vi "Main.vi"(11 "Module Admin":refnum<class "Delacor_lib_QMH_Module Admin.lvclass">) -> ()   [LabVIEW 2024, in "UIs Handler.lvlib"]
doc: "This template is based off of the Queued Message Handler design pattern and the Queued Message Handler project template that ships with LabVIEW.\n\nThe main difference is that the queue is private to this module and communication between modules is performed via Broadcast and Request events.\n\nRequest events are wrapped in public API methods and are handled in the Event Handling Loop (EHL) of this VI. Any module can register for Broadcast events sent by this module. The EHL generates messages based on user interface actions.\n\nThe Message Handling Loop (MHL) processes messages generated by the EHL, or by other messages. The messages are string values, so new messages can be added easily to the Message Cases case structure in the MHL. Each message cluster can also provide an optional value for Message Data, which is a variant that can be converted to whatever message-specific data is required.\n_____\nBased on DQMH Dev Tools: Project Template 7.1.0.1490."
uses:
  UIs Handler.lvlib
  <vilib>/Delacor/Delacor QMH/Libraries/Module Admin_class/Delacor_lib_QMH_Module Admin.lvclass
  Module Data--cluster.ctl
  Stop Argument--cluster.ctl
  <vilib>/Delacor/Delacor QMH/Libraries/Message Queue_class/Delacor_lib_QMH_Message Queue.lvclass/Delacor_lib_QMH_Message Queue.ctl
  <vilib>/Delacor/Delacor QMH/Libraries/Module Admin_class/Delacor_lib_QMH_Module Admin.lvclass/Delacor_lib_QMH_Module Admin.ctl
  Insert UI into subpanel Argument--cluster.ctl
  UIs/Select UI.ctl
  Start Counter Argument--cluster.ctl
  Save Counter Argument--cluster.ctl
  <vilib>/Utility/miscctls.llb/LVPointTypeDef.ctl
  <vilib>/numeric/Random Number (Range) DBL.vi
  d7337ac3-38f4-4494-95c6-09e6596b0280.vi
  <vilib>/GPower/Timing/Library/Elapsed/Elapsed_ms.vi
  <vilib>/Delacor/Delacor QMH/Libraries/Message Queue_class/Delacor_lib_QMH_Enqueue Message (Single).vi
  <vilib>/Delacor/Delacor QMH/Libraries/Module Admin_class/Delacor_lib_QMH_Get External Launch.vi
  UIs/Dashboard.vi
  UIs/MetaTabs.vi
  <vilib>/GPower/VILauncher/Library/Open/OpenByRefnumAndRunFP.vi
  <vilib>/Utility/file.llb/Application Directory.vi
  <userlib>/_MGI/File/MGI Create Directory Chain.vi
  <vilib>/Utility/file.llb/Write Delimited Spreadsheet (DBL).vi
  <vilib>/Delacor/Delacor QMH/Libraries/Message Queue_class/Delacor_lib_QMH_Message Queue.lvclass
  <vilib>/GPower/Timing/GPTiming.lvlib
  <vilib>/GPower/VILauncher/VILauncher.lvlib
panel:
  out "file path":path
  out "Elapsed time":i32 caption="Elapsed time [ms]"
  out "output cluster":T1
  out "Waveform Chart":T2(graph)
  out "error out":errorcluster
  out "Status":string
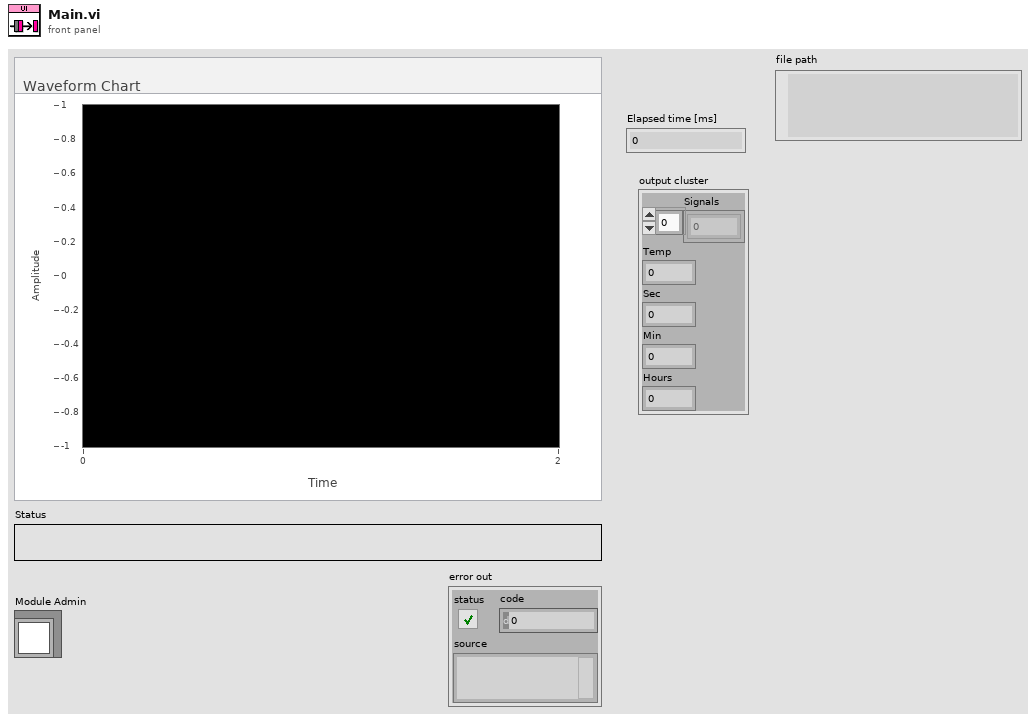
[diagram p1: front panel]
types:
  T1 = cluster{"Signals":dbl[], "Temp":dbl, "Sec":i32, "Min":i32, "Hours":i32}
  T2 = cluster{"shuffled array[0]":dbl, "shuffled array[1]":dbl, "shuffled array[2]":dbl, "shuffled array[3]":dbl, "shuffled array[4]":dbl, "shuffled array[5]":dbl, "shuffled array[6]":dbl, "shuffled array[7]":dbl, "shuffled array[8]":dbl, "shuffled array[9]":dbl, "shuffled array[10]":dbl, "shuffled array[11]":dbl, "shuffled array[12]":dbl, "shuffled array[13]":dbl, "shuffled array[14]":dbl, "shuffled array[15]":dbl, "shuffled array[16]":dbl, "shuffled array[17]":dbl, "shuffled array[18]":dbl, "shuffled array[19]":dbl}
  T3 = typedef "UIs Handler.lvlib/Request Events--cluster.ctl" = cluster{"Stop Module":refnum<user-event>, "Show Panel":refnum<user-event>, "Hide Panel":refnum<user-event>, "Get Module Execution Status":refnum<user-event>, "Show Diagram":refnum<user-event>, "Insert UI into subpanel":refnum<user-event>, "Start Counter":refnum<user-event>, "Reset Counter":refnum<user-event>, "Save Counter":refnum<user-event>, "Dashboard HLwakeup":refnum<user-event>, "Start Dashboard Monitoring":refnum<user-event>}
  T4 = typedef "UIs Handler.lvlib/Module Data--cluster.ctl" = cluster{"Status":string}
  T5 = cluster{"shuffled array[0]":dbl, "shuffled array[1]":dbl, "shuffled array[2]":dbl, "shuffled array[3]":dbl, "shuffled array[4]":dbl, "shuffled array[5]":dbl, "shuffled array[6]":dbl, "shuffled array[7]":dbl, "shuffled array[8]":dbl, "shuffled array[9]":dbl, "shuffled array[10]":dbl, "shuffled array[11]":dbl, "shuffled array[12]":dbl, "shuffled array[13]":dbl, "shuffled array[14]":dbl, "shuffled array[15]":dbl, "shuffled array[16]":dbl, "shuffled array[17]":dbl, "shuffled array[18]":dbl, "shuffled array[19]":dbl}[]
  T6 = enum32{"invalid lock state", "Not Locked", "Locked (No Password)", "Password-protected"}
  T7 = typedef "UIs Handler.lvlib/Stop Argument--cluster.ctl" = cluster{"Origin":string, "Exit via Stop Module Req?":bool, "Wait for Module to stop?":bool}
  T8 = typedef "UIs Handler.lvlib/Insert UI into subpanel Argument--cluster.ctl" = cluster{"Subpanel":refnum<vi>, "Select UI":T9}
  T9 = typedef "UIs Handler.lvlib/Select UI.ctl" = enum16{"Dashboard", "Meta Tabs"}
  T10 = typedef "UIs Handler.lvlib/Start Counter Argument--cluster.ctl" = cluster{"Boolean":bool}
  T11 = typedef "UIs Handler.lvlib/Save Counter Argument--cluster.ctl" = cluster{"Boolean":bool}
  T12 = typedef "LVPointTypeDef.ctl" = cluster{"Horizontal":i16, "Vertical":i16}
  T13 = enum32{"Invalid", "Standard", "Closed", "Hidden", "Minimized", "Maximized"}
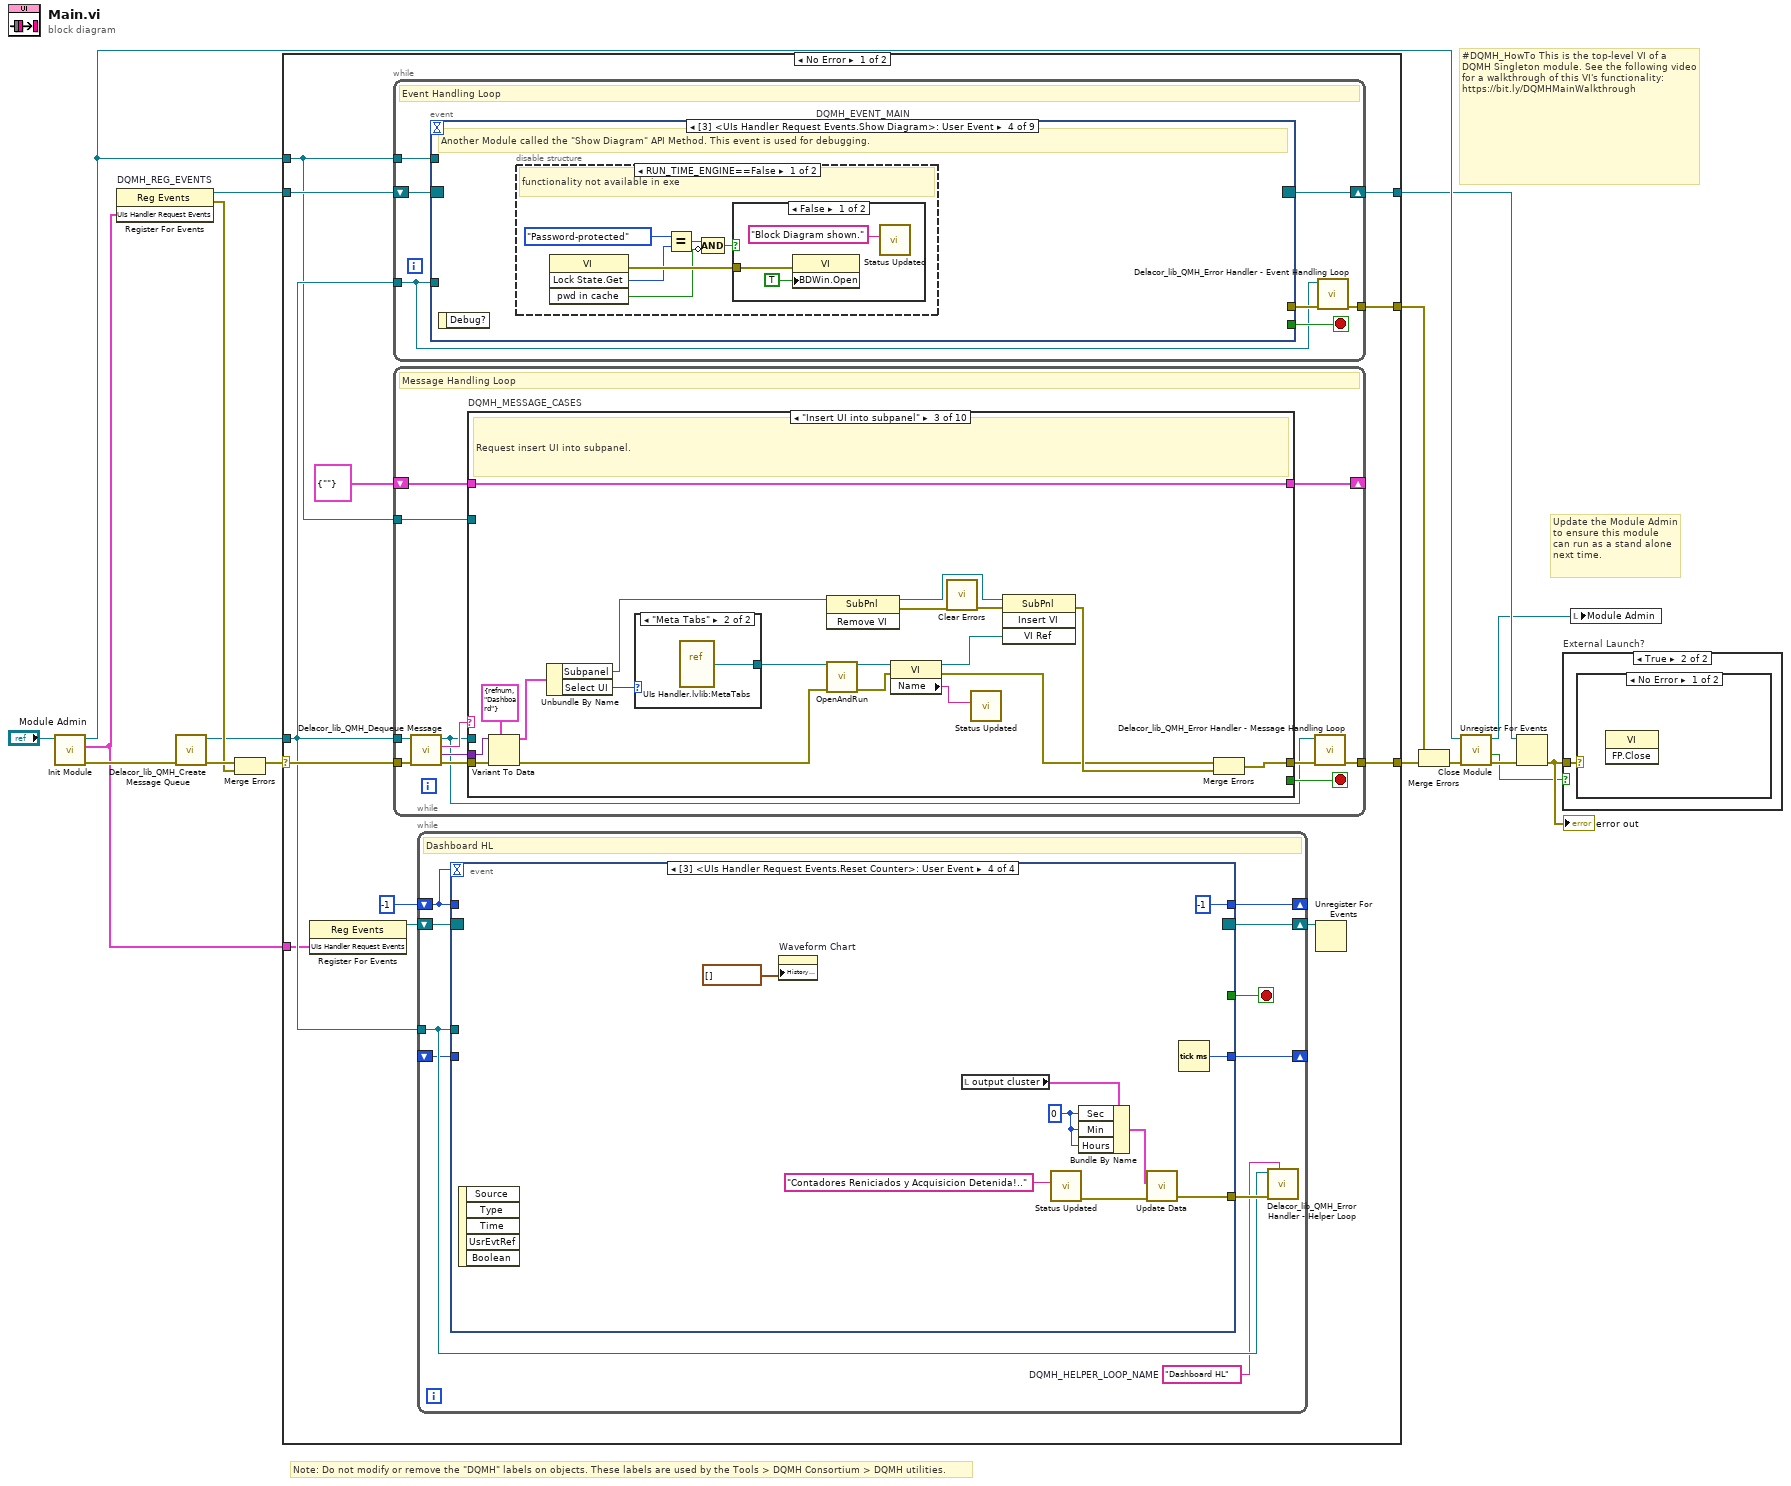
[diagram p0: block diagram]
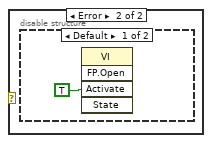
[diagram p3: hidden frame]
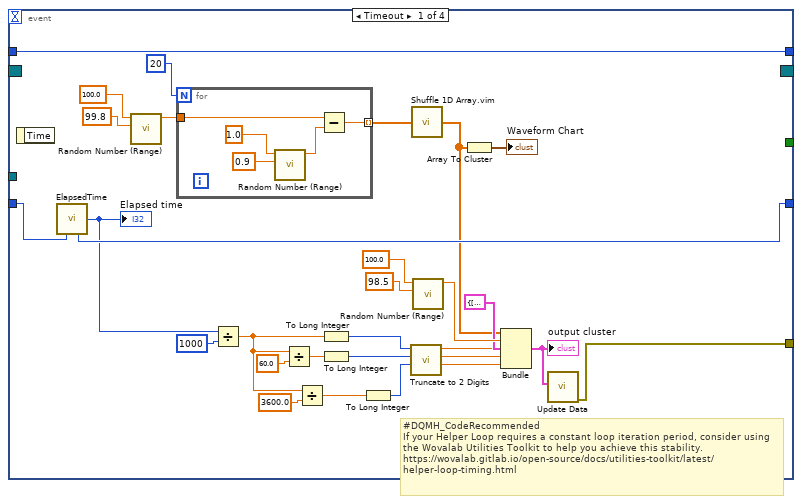
[diagram p5: hidden frame]
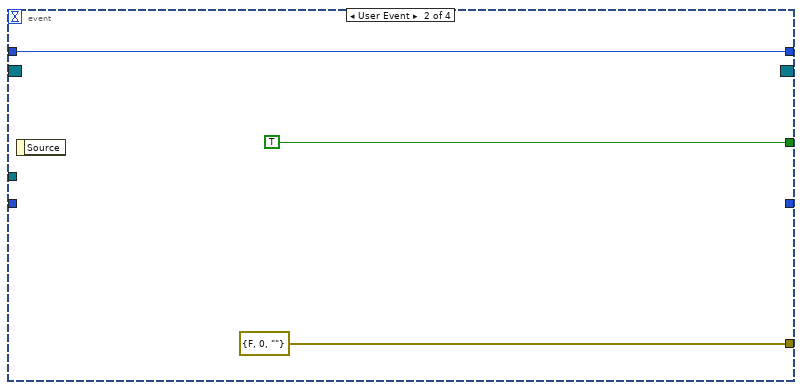
[diagram p6: hidden frame]
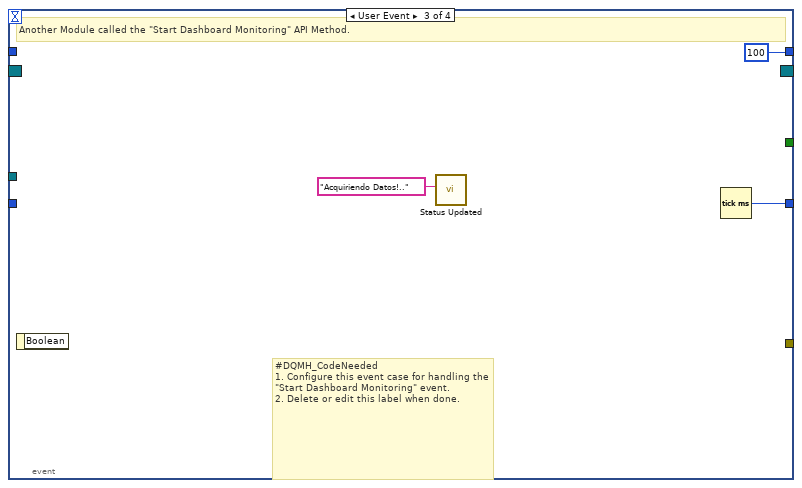
[diagram p7: hidden frame]
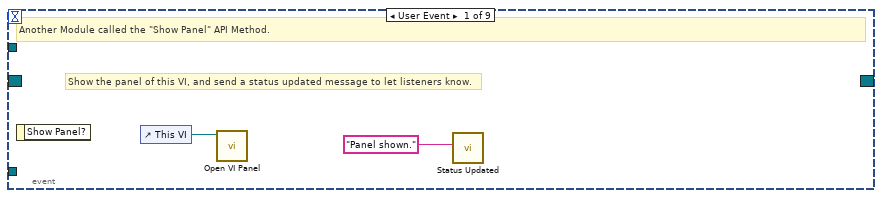
[diagram p8: hidden frame]
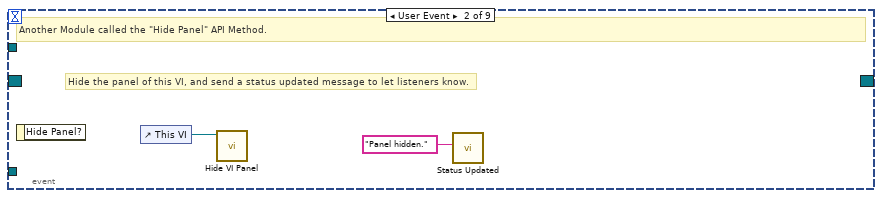
[diagram p9: hidden frame]
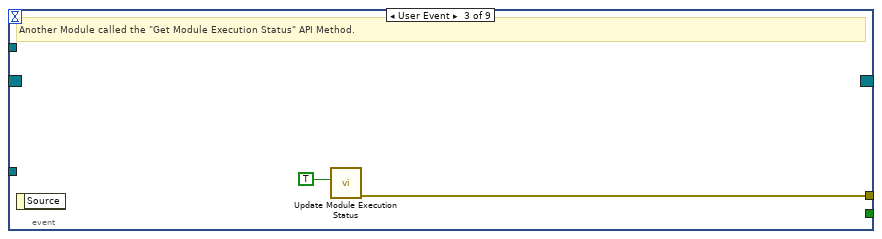
[diagram p10: hidden frame]
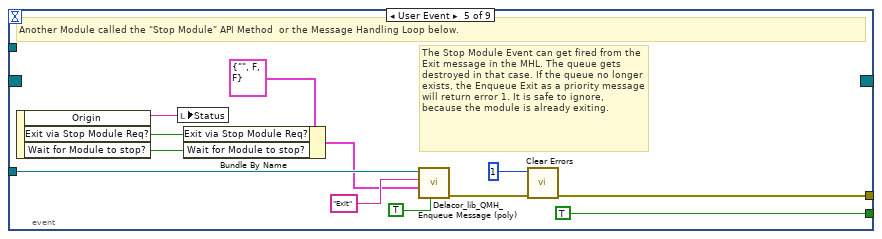
[diagram p13: hidden frame]
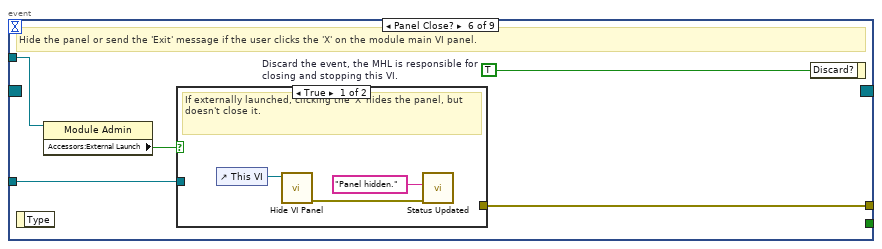
[diagram p14: hidden frame]
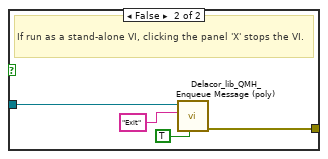
[diagram p15: hidden frame]
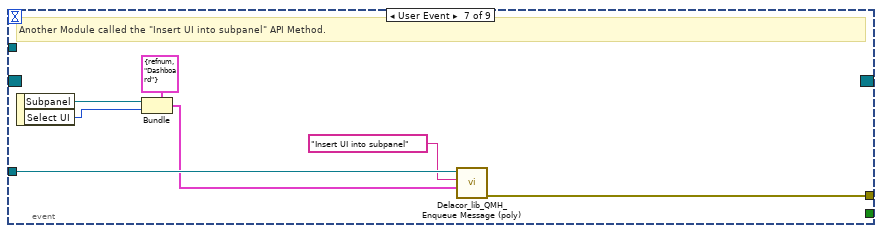
[diagram p16: hidden frame]
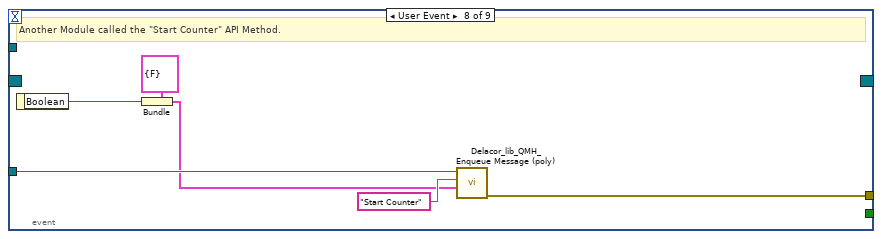
[diagram p17: hidden frame]
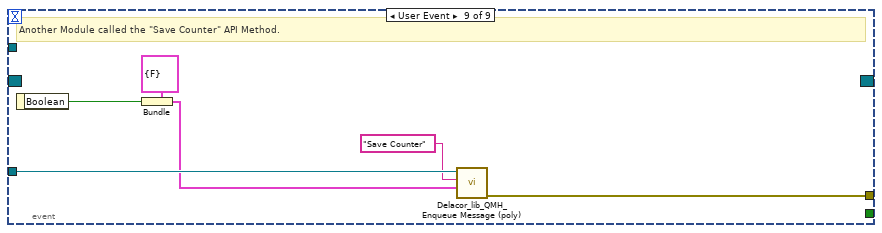
[diagram p18: hidden frame]
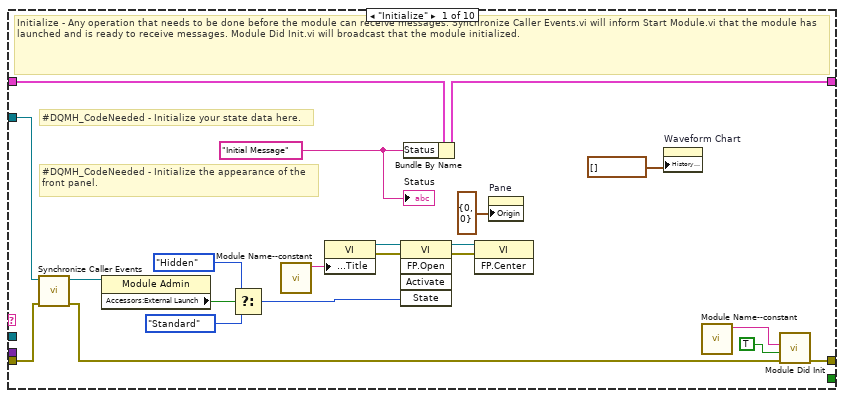
[diagram p19: hidden frame]
diagram:
  # "#DQMH_HowTo This is the top-level VI of a DQMH Singleton module. See the following video for a walkthrough of this VI's functionality: https://bit.ly/DQMHMainWalkthrough"
  # "Note: Do not modify or remove the \"DQMH\" labels on objects. These labels are used by the Tools > DQMH Consortium > DQMH utilities."
  # "Update the Module Admin to ensure this module can run as a stand alone next time."
  n1 = call "Init Module.vi"("Singleton Module Admin in"="Module Admin") -> ("error out"=w16:errorcluster, "UIs Handler Request Events"=w1:T3, "Singleton Module Admin out"=w8:refnum<class "Delacor_lib_QMH_Module Admin.lvclass">)  [unwired: 8 in]
  n2 = register-events "DQMH_REG_EVENTS"(w1) -> (reference out=w6:refnum<event-registration>, error out=w9:errorcluster)  [unwired: 2 in]
  n3 = call <vilib>:"Delacor_lib_QMH_Create Message Queue.vi"("error in"=w16) -> ("error out"=w11:errorcluster, "Message Queue"=w5:refnum<class "Delacor_lib_QMH_Message Queue.lvclass">)  [unwired: 9 in]
  n4 = Merge Errors(w11, w9) -> (w10:errorcluster)
  n5 = case shown="No Error" w10 {
    selector: w10 -> [w27 w288]
    tunnel: [w29 w287] -> w17
    tunnel: [w26 w286] -> w7
    tunnel: w6 -> [w24 w286]
    tunnel: w5 -> [w23 w281]
    tunnel: [w28 _] -> w14
    tunnel: w8 -> [w22 w282]
    tunnel: w1 -> [w21 _]
    frame No Error {
      n6 = register-events ("DQMH_HELPER_REGFOREVENTS")(w21) -> (reference out=w19:refnum<event-registration>)  [unwired: 2 in, 1 out]
      n7 = while {
        tunnel: w23 -> [w89]
        shift-right: [w92] -> w26
        shift-left: w24 -> [w93]
        tunnel: [w94] -> w28
        tunnel: w22 -> [w90]
        stop <- w91 stop-if-true
        # "Event Handling Loop"
        n8 = event "DQMH_EVENT_MAIN" shown="[3] <UIs Handler Request Events.Show Diagram>: User Event" {
          selector: w93 -> [_ _ _ _ _ _ _ _ _]
          dyn-events: [_ _ _ _ _ _ _ _ _] -> w92
          timeout: _ -> [_ _ _ _ _ _ _ _ _]
          tunnel: [_ _ _ _ TRUE ("Discard?") _ _ _ _] -> w91
          tunnel: w89 -> [_ _ _ _ w118 w125 w141 w147 w153]
          tunnel: [_ _ w101 _ w121 w127 w135 w142 w148] -> w95
          tunnel: w90 -> [_ _ _ _ _ w124 _ _ _]
          event User Event {
            # "Show the panel of this VI, and send a status updated message to let listeners know."
            # "Another Module called the \"Show Panel\" API Method."
            n9 = event-data() -> ()  [unwired: 1 in, 1 out]
            n10 = control-ref of="This VI"() -> (w97:refnum<vi>)
            n11 = call "Open VI Panel.vi"("VI"=w97) -> ()  [unwired: 10 in, 1 out]
            n12 = call "Status Updated.vi"("Status"="Panel shown." ("format string")) -> ()  [unwired: 10 in, 1 out]
          }
          event User Event {
            # "Hide the panel of this VI, and send a status updated message to let listeners know."
            # "Another Module called the \"Hide Panel\" API Method."
            n13 = event-data() -> ()  [unwired: 1 in, 1 out]
            n14 = control-ref of="This VI"() -> (w99:refnum<vi>)
            n15 = call "Hide VI Panel.vi"("VI"=w99) -> ()  [unwired: 10 in, 1 out]
            n16 = call "Status Updated.vi"("Status"="Panel hidden." ("format string")) -> ()  [unwired: 10 in, 1 out]
          }
          event User Event {
            # "Another Module called the \"Get Module Execution Status\" API Method."
            n17 = event-data() -> ()  [unwired: 1 in, 1 out]
            n18 = call "Update Module Execution Status.vi"("Running?"=TRUE) -> ("error out"=w101:errorcluster)  [unwired: 10 in]
          }
          event User Event {
            # "Another Module called the \"Show Diagram\" API Method. This event is used for debugging."
            n19 = event-data() -> ()  [unwired: 1 in, 1 out]
            n20 = disable-structure shown="RUN_TIME_ENGINE==False" {
              frame condition #0 (active) {
                # "functionality not available in exe"
                n21 = invoke on="Invoke Node" class="VI" method="Lock State.Get"() -> (error out=w107:errorcluster, "Get Lock State"=w106:T6, "pwd in cache"=w103:bool)  [unwired: 4 in, 1 out]
                n22 = Equal?(x=T6."Password-protected", y=w106) -> (x = y?=w104:bool)
                n23 = Compound Arithmetic op=AND(w104, invert w103) -> (w102:bool)
                n24 = case shown="False" w102 {
                  tunnel: w107 -> [w110 _]
                  frame False {
                    n25 = property on="Property Node" class="VI"(error in=w110, "BDWin.Open"=TRUE ("Block Diagram Window:Open")) -> ()  [unwired: 1 in, 2 out]
                    n26 = call "Status Updated.vi"("Status"="Block Diagram shown." ("format string")) -> ()  [unwired: 10 in, 1 out]
                  }
                  frame True {
                    # "Password-protected VI, and the password is not in the cache. Do not show the diagram."
                  }
                }
              }
              frame condition #1 {
              }
            }
          }
          event User Event {
            # "The Stop Module Event can get fired from the Exit message in the MHL. The queue gets destroyed in that case. If the queue no longer exists, the Enqueue Exit as a priority message will return error 1. It is safe to ignore, because the module is already exiting."
            # "Another Module called the \"Stop Module\" API Method  or the Message Handling Loop below."
            n27 = event-data() -> ("Origin"=w117:string, "Exit via Stop Module Req?"=w113:bool, "Wait for Module to stop?"=w112:bool)  [unwired: 1 in]
            n28 = local write "Status"(w117) -> ()
            n29 = Bundle By Name(cluster=T7 {"Origin"="", "Exit via Stop Module Req?"=FALSE, "Wait for Module to stop?"=FALSE} ("Stop Argument"), "Exit via Stop Module Req?"=w113, "Wait for Module to stop?"=w112) -> (w111:T7)
            n30 = call-poly <vilib>:"Delacor_lib_QMH_Enqueue Message (poly).vi"("Priority Message? (F)"=TRUE, "Message Data"=w111, "Message"="Exit", "Message Queue in"=w118) -> ("error out"=w122:errorcluster)  [unwired: 6 in, 1 out]
            n31 = call <vilib>:"Clear Errors.vi"("error in (no error)"=w122, "specific error code to clear (0: all)"=1) -> ("error out"=w121:errorcluster)  [unwired: 4 in, 1 out]
          }
          event Panel Close? {
            w126 = TRUE  # Discard the event, the MHL is responsible for closing and stopping this VI.
            # "Hide the panel or send the 'Exit' message if the user clicks the 'X' on the module main VI panel."
            n32 = event-data() -> ()  [unwired: 1 in, 1 out]
            n33 = property on="Property Node" class="Module Admin"(reference=w124) -> ("Accessors:External Launch"=w123:bool)  [unwired: 1 in, 2 out]
            n34 = case shown="True" w123 {
              tunnel: w125 -> [_ w133]
              tunnel: [_ w134] -> w127
              frame True {
                # "If externally launched, clicking the 'X' hides the panel, but doesn't close it."
                n35 = control-ref of="This VI"() -> (w130:refnum<vi>)
                n36 = call "Hide VI Panel.vi"("VI"=w130) -> ("error out"=w128:errorcluster)  [unwired: 10 in]
                n37 = call "Status Updated.vi"("error in"=w128, "Status"="Panel hidden." ("format string")) -> ()  [unwired: 9 in, 1 out]
              }
              frame False {
                # "If run as a stand-alone VI, clicking the panel 'X' stops the VI."
                n38 = call-poly <vilib>:"Delacor_lib_QMH_Enqueue Message (poly).vi"("Priority Message? (F)"=TRUE, "Message"="Exit", "Message Queue in"=w133) -> ("error out"=w134:errorcluster)  [unwired: 7 in, 1 out]
              }
            }
            n39 = event-data ("Event Filter Node")("Discard?"=w126) -> ()  [unwired: 1 in, 1 out]
          }
          event User Event {
            # "Another Module called the \"Insert UI into subpanel\" API Method."
            n40 = event-data() -> ("Subpanel"=w137:refnum<vi>, "Select UI"=w136:T9)  [unwired: 1 in]
            n41 = Bundle(cluster=T8 {"Subpanel"=refnum, "Select UI"=enum."Dashboard"} ("Insert UI into subpanel Argument"), "Subpanel"=w137, "Select UI"=w136) -> (w138:T8)
            n42 = call-poly <vilib>:"Delacor_lib_QMH_Enqueue Message (poly).vi"("Message Data"=w138, "Message"="Insert UI into subpanel", "Message Queue in"=w141) -> ("error out"=w135:errorcluster)  [unwired: 7 in, 1 out]
          }
          event User Event {
            # "Another Module called the \"Start Counter\" API Method."
            n43 = event-data() -> ("Boolean"=w143:bool)  [unwired: 1 in]
            n44 = Bundle(cluster=T10 {"Boolean"=FALSE} ("Start Counter Argument"), "Boolean"=w143) -> (w144:T10)
            n45 = call-poly <vilib>:"Delacor_lib_QMH_Enqueue Message (poly).vi"("Message Data"=w144, "Message"="Start Counter", "Message Queue in"=w147) -> ("error out"=w142:errorcluster)  [unwired: 7 in, 1 out]
          }
          event User Event {
            # "Another Module called the \"Save Counter\" API Method."
            n46 = event-data() -> ("Boolean"=w149:bool)  [unwired: 1 in]
            n47 = Bundle(cluster=T11 {"Boolean"=FALSE} ("Save Counter Argument"), "Boolean"=w149) -> (w150:T11)
            n48 = call-poly <vilib>:"Delacor_lib_QMH_Enqueue Message (poly).vi"("Message Data"=w150, "Message"="Save Counter", "Message Queue in"=w153) -> ("error out"=w148:errorcluster)  [unwired: 7 in, 1 out]
          }
        }
        n49 = call-dynamic "Delacor_lib_QMH_Error Handler - Event Handling Loop.vi"("error in"=w95, "Message Queue in"=w89) -> ("dup error in"=w94:errorcluster)  [unwired: 8 in, 1 out]
      }
      n50 = while {
        tunnel: w23 -> [w154]
        shift-right: [w162] -> _
        shift-left: T4 {"Status"=""} ("Data Cluster") -> [w163]
        tunnel: w27 -> [w165]
        tunnel: [w157] -> w29
        tunnel: w22 -> [w158]
        stop <- w161 stop-if-true
        # "Message Handling Loop"
        n51 = call-dynamic "Delacor_lib_QMH_Dequeue Message.vi"("error in"=w165, "Message Queue in"=w154) -> ("error out"=w164:errorcluster, "Message Data"=w159:variant, "Message"=w160:string, "Message Queue out"=w155:refnum<class "Delacor_lib_QMH_Message Queue.lvclass">)  [unwired: 6 in]
        n52 = case "DQMH_MESSAGE_CASES" shown="\"Insert UI into subpanel\"" w160 {
          selector: w160 -> [_ _ _ _ _ _ _ _ _ w276]
          tunnel: w155 -> [_ _ _ _ _ _ _ w242 w264 _]
          tunnel: w164 -> [w184 w188 w207 w217 w233 w236 w238 w249 w270 w279]
          tunnel: [w182 w188 w195 w210 w221 w235 w238 w245 w265 w280] -> w156
          tunnel: w163 -> [w173 w187 w206 w216 w232 w234 w237 w244 w263 w277]
          tunnel: [w172 w187 w206 w216 w232 w234 w237 w244 w263 w277] -> w162
          tunnel: [_ _ _ _ _ _ _ _ w262 _] -> w161
          tunnel: w159 -> [_ _ w205 w215 w231 _ _ w243 w261 _]
          tunnel: w158 -> [w174 _ _ _ _ _ _ w241 w256 _]
          frame "Initialize" {
            w168 = "Initial Message" ("Initial Message")
            # "#DQMH_CodeNeeded - Initialize the appearance of the front panel."
            # "#DQMH_CodeNeeded - Initialize your state data here."
            # "Initialize - Any operation that needs to be done before the module can receive messages. Synchronize Caller Events.vi will inform Start Module.vi that the module has launched and is ready to receive messages. Module Did Init.vi will broadcast that the module initialized."
            n53 = call "Synchronize Caller Events.vi"("error in"=w184, "Singleton Module Admin in"=w174) -> ("error out"=w183:errorcluster, "Singleton Module Admin out"=w169:refnum<class "Delacor_lib_QMH_Module Admin.lvclass">)  [unwired: 8 in]
            n54 = property on="Property Node" class="Module Admin"(reference=w169) -> ("Accessors:External Launch"=w178:bool)  [unwired: 1 in, 2 out]
            n55 = Select(t=T13."Hidden" ("State"), s=w178, f=T13."Standard" ("State")) -> (s? t:f=w175:T13)
            n56 = call "Module Name--constant.vi"() -> ("Module Name"=w181:string)  [unwired: 11 in]
            n57 = property on="Property Node" class="VI"("Front Panel.Title"=w181) -> (reference out=w180:refnum<vi>, error out=w186:errorcluster)  [unwired: 2 in]
            n58 = invoke on="Invoke Node" class="VI" method="FP.Open"(reference=w180, error in=w186, "State"=w175) -> (reference out=w179:refnum<vi>, error out=w185:errorcluster)  [unwired: 2 in, 3 out]
            n59 = Bundle By Name(cluster=w173, "Status"=w168) -> (w172:T4)
            n60 = invoke on="Invoke Node" class="VI" method="FP.Center"(reference=w179, error in=w185) -> ()  [unwired: 1 in, 3 out]
            n61 = property on="Pane" class="Pane"("Origin"=T12 {"Horizontal"=0, "Vertical"=0}) -> ()  [unwired: 2 in, 2 out]
            n62 = property on="Waveform Chart" class="WFChart (strict)"("History Data"=T5 []) -> ()  [unwired: 2 in, 2 out]
            n63 = call "Module Name--constant.vi"() -> ("Module Name"=w170:string)  [unwired: 11 in]
            n64 = call "Module Did Init.vi"("error in"=w183, "Initialized?"=TRUE, "Origin"=w170) -> ("error out"=w182:errorcluster)  [unwired: 8 in]
            "Status" <- w168
          }
          frame "---Module Specific---" {
            # "Separator -- The following cases handle messages specific to this Module."
          }
          frame "Insert UI into subpanel" {
            # "Request insert UI into subpanel."
            n65 = Variant To Data(error in=w207, type=T8 {"Subpanel"=refnum, "Select UI"=enum."Dashboard"} ("Insert UI into subpanel Argument"), Variant=w205) -> (data=w203:T8, error out=w196:errorcluster)
            n66 = Unbundle By Name(w203) -> ("Subpanel"=w201:refnum<vi>, "Select UI"=w202:T9)
            n67 = case shown="\"Meta Tabs\"" w202 {
              tunnel: [w208 w209] -> w197
              frame "Dashboard", Default {
                n68 = vi-ref "UIs Handler.lvlib:Dashboard.vi"() -> (w208:refnum<vi>)
              }
              frame "Meta Tabs" {
                n69 = vi-ref "UIs Handler.lvlib:MetaTabs.vi"() -> (w209:refnum<vi>)
              }
            }
            n70 = invoke on="Invoke Node" class="SubPnl" method="Remove VI"(reference=w201) -> (reference out=w198:refnum<vi>, error out=w199:errorcluster)  [unwired: 2 in, 1 out]
            n71 = call-poly <vilib>:"OpenAndRun.vi"("VI refnum"=w197, "Error in"=w196) -> ("VI refnum out"=w193:refnum<vi>, "Error out"=w191:errorcluster)  [unwired: 7 in, 5 out]
            n72 = property class="VI"(reference=w193, error in=w191) -> (reference out=w192:refnum<vi>, error out=w190:errorcluster, "Name"=w189:string)
            n73 = call <vilib>:"Clear Errors.vi"("error in (no error)"=w199) -> ("error out"=w200:errorcluster)  [unwired: 5 in, 1 out]
            n74 = call "Status Updated.vi"("Status"=w189) -> ()  [unwired: 10 in, 1 out]
            n75 = invoke on="Invoke Node" class="SubPnl" method="Insert VI"(reference=w198, error in=w200, "VI Ref"=w192) -> (error out=w194:errorcluster)  [unwired: 1 in, 3 out]
            n76 = Merge Errors(w190, w194) -> (w195:errorcluster)
          }
          frame "Start Counter" {
            # "Start Counter"
            n77 = Variant To Data(error in=w217, type=T10 {"Boolean"=FALSE} ("Start Counter Argument"), Variant=w215) -> (data=w213:T10, error out=w211:errorcluster)
            n78 = Unbundle By Name(w213) -> ()  [unwired: 1 out]
            n79 = call "Start Dashboard Monitoring.vi"("error in"=w211) -> ("error out"=w210:errorcluster)  [unwired: 10 in]
            n80 = call "Status Updated.vi"("Status"="Counter Started!..") -> ()  [unwired: 10 in, 1 out]
          }
          frame "Save Counter" {
            # "Save Counter"
            n81 = Variant To Data(error in=w233, type=T11 {"Boolean"=FALSE} ("Save Counter Argument"), Variant=w231) -> (data=w229:T11, error out=w226:errorcluster)
            n82 = Unbundle By Name(w229) -> ()  [unwired: 1 out]
            n83 = local read "Waveform Chart"() -> (w224:T2)
            n84 = call "Datalogger Path--constant.vi"("Error In"=w226) -> ("Error Out"=w227:errorcluster, "Path"=w225:path)  [unwired: 9 in]
            n85 = Cluster To Array(cluster=w224) -> (array=w223:dbl[])
            n86 = call-poly <vilib>:"Write Delimited Spreadsheet.vi"("file path (dialog if empty)"=w225, "1D data"=w223, "error in (no error)"=w227) -> ("new file path (Not A Path if cancelled)"=→"file path":path, "error out"=w221:errorcluster)  [unwired: 11 in]
            n87 = Not(x=w221) -> (.not. x?=w220:bool)
            n88 = Select(t="Datos Salvados!.." ("Status"), s=w220, f="Error Tratando de salvar datos!.." ("Status")) -> (s? t:f=w218:string)
            n89 = call "Status Updated.vi"("Status"=w218) -> ()  [unwired: 10 in, 1 out]
          }
          frame "---Copy This Frame---" {
            # "Duplicate this frame when creating new messages.  Change this comment in the duplicated frame to describe this message."
            n90 = Merge Errors(w236) -> (w235:errorcluster)
          }
          frame "---Exit and Error Handling---" {
            # "Separator - The following cases handle errors and exit messages."
          }
          frame "Error" {
            # "#DQMH_CodeRecommended - If the module is running in standalone mode (External Launch = FALSE), this code will pop up an error dialog and call the 'Exit' message if an error occurs. Add more fine-grained error management here."
            # "Error - Check the error message data and respond accordingly. This message is sent by the \"Error Handler\" VIs at the end of each loop in this application."
            n91 = property on="Property Node" class="Module Admin"(reference=w241) -> ("Accessors:External Launch"=w240:bool)  [unwired: 1 in, 2 out]
            n92 = Variant To Data(error in=w249, type=errorcluster {"status"=FALSE, "code"=0, "source"=""} ("error constant"), Variant=w243) -> (data=w239:errorcluster, error out=w247:errorcluster)
            n93 = local write "error out"(w239) -> ()
            n94 = call "Error Reported.vi"("Error"=w239) -> ()  [unwired: 10 in, 1 out]
            n95 = case shown="False" w240 {
              tunnel: [w254 _] -> w246
              tunnel: w242 -> [w252 _]
              tunnel: w239 -> [w253 _]
              frame False {
                n96 = disable-structure shown="Default" {
                  disable-tunnel: w253 -> [w255 _]
                  frame condition #0 (active) {
                    # "If the module is running standalone, then pop up an error dialog and call the \"Exit\" message."
                    n97 = call <vilib>:"Simple Error Handler.vi"("error in (no error)"=w255) -> ()  [unwired: 4 in, 5 out]
                  }
                  frame condition #1 {
                    # "To prevent the Simple Error Handler VI from being loaded (e.g. when deploying to a Real-Time target), add the Conditional Disable Symbol \"DQMH_Disable_SEH\" to your project and set it to TRUE."
                  }
                }
                n98 = call-poly <vilib>:"Delacor_lib_QMH_Enqueue Message (poly).vi"("Priority Message? (F)"=TRUE, "Message"="Exit", "Message Queue in"=w252) -> ("error out"=w254:errorcluster)  [unwired: 7 in, 1 out]
              }
              frame True {
                # "If the module was launched externally, calling the Error Reported broadcast VI is the only action performed by the \"Error\" message. The module's caller can then process the error appropriately."
              }
            }
            n99 = Merge Errors(w247, w246) -> (w245:errorcluster)
          }
          frame "Exit" {
            w260 = 91  # 91: not all Exit messages will have an argument
            w262 = TRUE  # Stop the VI
            # "Release the message queue reference"
            # "#DQMH_CodeNeeded - Add any required cleanup code here."
            # "Exit - Exit the application."
            n100 = Variant To Data(error in=w270, type=T7 {"Origin"="", "Exit via Stop Module Req?"=FALSE, "Wait for Module to stop?"=FALSE} ("Stop Argument"), Variant=w261) -> (data=w258:T7, error out=w267:errorcluster)
            n101 = call <vilib>:"Clear Errors.vi"("error in (no error)"=w267, "specific error code to clear (0: all)"=w260) -> ("error out"=w269:errorcluster)  [unwired: 4 in, 1 out]
            n102 = control-ref of="This VI"() -> (w257:refnum<vi>)
            n103 = call-dynamic "Delacor_lib_QMH_Release Message Queue.vi"("error in"=w269, "Message Queue"=w264) -> ("error out"=w268:errorcluster)  [unwired: 9 in]
            n104 = call "Handle Exit.vi"("Stop Argument"=w258, "Admin in"=w256, "VI reference"=w257) -> ("error out"=w266:errorcluster)  [unwired: 7 in, 1 out]
            n105 = Merge Errors(w268, w266) -> (w265:errorcluster)
            n106 = call "Error Reported.vi"("Error"=w265) -> ()  [unwired: 10 in, 1 out]
          }
          frame Default {
            # "'Default' case only runs if there is a message that isn't defined in any of the other cases.  Output a programming error."
            n107 = call "Module Name--constant.vi"() -> ("Module Name"=w275:string)  [unwired: 11 in]
            n108 = Format Into String(format string="The invalid message string \"%s\" was received in the Message Handling Loop for module \"%s\".", w276, w275) -> (resulting string=w271:string)  [unwired: 2 in, 1 out]
            n109 = call <vilib>:"Error Cluster From Error Code.vi"("show call chain? (False)"=TRUE, "error message (\"\")"=w271, "error code (0)"=1) -> ("error out"=w278:errorcluster)  [unwired: 6 in]
            n110 = Merge Errors(w279, w278) -> (w280:errorcluster)
          }
        }
        n111 = call-dynamic "Delacor_lib_QMH_Error Handler - Message Handling Loop.vi"("error in"=w156, "Message Queue in"=w155) -> ("dup error in"=w157:errorcluster)  [unwired: 8 in, 1 out]
      }
      n112 = while "DQMH_HELPER_LOOP" {
        shift-right: [w39] -> _
        shift-left: -1 -> [w38]
        shift-right: [w36] -> w20
        shift-left: w19 -> [w37]
        tunnel: w23 -> [w33]
        shift-right: [w31] -> _
        shift-left: _ -> [w30]
        stop <- w35 stop-if-true
        w32 = "Dashboard HL"  # DQMH_HELPER_LOOP_NAME
        # "Dashboard HL"
        n113 = event "DQMH_HELPER_EVENT_STRUCTURE" shown="[3] <UIs Handler Request Events.Reset Counter>: User Event" {
          selector: w37 -> [_ _ _ _]
          dyn-events: [_ _ _ _] -> w36
          timeout: w38 -> [_ _ _ _]
          tunnel: w38 -> [w68 w76 _ _]
          tunnel: [w68 w76 100 -1] -> w39
          tunnel: [_ TRUE _ _] -> w35
          tunnel: [w53 errorcluster {"status"=FALSE, "code"=0, "source"=""} ("error constant") _ w80] -> w34
          tunnel: w33 -> [_ _ _ _]
          tunnel: [w63 _ w78 w88] -> w31
          tunnel: w30 -> [w64 _ _ _]
          event Timeout {
            # "#DQMH_CodeRecommended\nIf your Helper Loop requires a constant loop iteration period, consider using the Wovalab Utilities Toolkit to help you achieve this stability.\nhttps://wovalab.gitlab.io/open-source/docs/utilities-toolkit/latest/helper-loop-timing.html"
            n114 = event-data() -> ()  [unwired: 1 in, 1 out]
            n115 = call-poly <vilib>:"ElapsedTime.vi"("Start time in"=w64) -> ("Elapsed time"=w52:i32, "Start time out"=w63:i64)  [unwired: 11 in, 2 out]
            "Elapsed time" <- w52
            n116 = call-poly <vilib>:"Random Number (Range).vi"("lower bound (0)"=99.8, "upper bound (100)"=100.0) -> ("number"=w49:dbl)  [unwired: 9 in]
            n117 = for {
              N: 20 -> [_]
              tunnel: w49 -> [w72]
              tunnel: [w73] -> w47 mode=indexing
              n118 = call-poly <vilib>:"Random Number (Range).vi"("lower bound (0)"=0.9, "upper bound (100)"=1.0) -> ("number"=w69:dbl)  [unwired: 9 in]
              n119 = Subtract(x=w72, y=w69) -> (x-y=w73:dbl)
            }
            n120 = Divide(x=w52, y=i64 1000) -> (x/y=w59:dbl)
            n121 = Divide(x=w59, y=60.0) -> (x/y=w57:dbl)
            n122 = Divide(x=w59, y=3600.0) -> (x/y=w56:dbl)
            n123 = To Long Integer(number=w59) -> (32bit integer=w45:i32)
            n124 = To Long Integer(number=w57) -> (32bit integer=w44:i32)
            n125 = To Long Integer(number=w56) -> (32bit integer=w43:i32)
            n126 = call "Truncate to 2 Digits.vi"("Hours In"=w43, "Minutes In"=w44, "Sec In"=w45) -> ("Hours Out"=w40:dbl, "Minutes Out"=w41:dbl, "Sec Out"=w42:dbl)  [unwired: 6 in]
            n127 = call "Shuffle 1D Array.vim"("array"=w47) -> ("shuffled array"=w46:dbl[])  [unwired: 4 in]
            n128 = call-poly <vilib>:"Random Number (Range).vi"("lower bound (0)"=98.5, "upper bound (100)"=100.0) -> ("number"=w61:dbl)  [unwired: 9 in]
            n129 = Array To Cluster(array=w46) -> (cluster=→"Waveform Chart":T2)
            n130 = Bundle(cluster=T1 {"Signals"=[], "Temp"=0.0, "Sec"=0, "Min"=0, "Hours"=0} ("output cluster"), "Signals"=w46, "Temp"=w61, "Sec"=w42, "Min"=w41, "Hours"=w40) -> (w54:T1)
            "output cluster" <- w54
            n131 = call "Update Data.vi"("output cluster"=w54) -> ("error out"=w53:errorcluster)  [unwired: 10 in]
          }
          event User Event {
            n132 = event-data() -> ()  [unwired: 1 in, 1 out]
          }
          event User Event {
            # "#DQMH_CodeNeeded\n1. Configure this event case for handling the \"Start Dashboard Monitoring\" event.\n2. Delete or edit this label when done."
            # "Another Module called the \"Start Dashboard Monitoring\" API Method."
            n133 = event-data() -> ()  [unwired: 1 in, 1 out]
            n134 = call "Status Updated.vi"("Status"="Acquiriendo Datos!..") -> ()  [unwired: 10 in, 1 out]
            n135 = Tick Count (ms)() -> (millisecond timer value=w78:u32)
          }
          event User Event {
            w83 = 0 ("Sec")
            n136 = event-data() -> ()  [unwired: 1 in, 5 out]
            n137 = property on="Waveform Chart" class="WFChart (strict)"("History Data"=T5 []) -> ()  [unwired: 2 in, 2 out]
            n138 = local read "output cluster"() -> (w81:T1)
            n139 = call "Status Updated.vi"("Status"="Contadores Reniciados y Acquisicion Detenida!..") -> ("error out"=w84:errorcluster)  [unwired: 10 in]
            n140 = Bundle By Name(cluster=w81, "Sec"=w83, "Min"=w83, "Hours"=w83) -> (w82:T1)
            n141 = call "Update Data.vi"("error in"=w84, "output cluster"=w82) -> ("error out"=w80:errorcluster)  [unwired: 9 in]
            n142 = Tick Count (ms)() -> (millisecond timer value=w88:u32)
          }
        }
        n143 = call-dynamic "Delacor_lib_QMH_Error Handler - Helper Loop.vi"("Error Debug"=w32, "error in"=w34, "Message Queue in"=w33) -> ()  [unwired: 7 in, 2 out]
      }
      n144 = Unregister For Events(event registration refnum=w20) -> ()  [unwired: 1 in, 1 out]
    }
    frame Error {
      # "Synchronize Caller Events.vi will inform Start Module.vi that the module has launched and will let the code calling Start Module.vi register for broadcasts and would permit the caller receive the broadcast that an error occurred at launch time."
      n145 = call-dynamic "Delacor_lib_QMH_Release Message Queue.vi"("error in"=w288, "Message Queue"=w281) -> ("error out"=w287:errorcluster)  [unwired: 9 in]
      n146 = call "Synchronize Caller Events.vi"("Singleton Module Admin in"=w282) -> ("error out"=w289:errorcluster)  [unwired: 9 in, 1 out]
      n147 = call "Module Name--constant.vi"() -> ("Module Name"=w285:string)  [unwired: 11 in]
      n148 = Format Into String(format string="An error occurred during initialization. %s is no longer running.", w285) -> (resulting string=w283:string)  [unwired: 2 in, 1 out]
      n149 = Merge Errors(w287, w289) -> (w290:errorcluster)
      n150 = call "Error Reported.vi"("Additional Information"=w283, "Error"=w290) -> ()  [unwired: 9 in, 1 out]
    }
  }
  n151 = Merge Errors(w14, w17) -> (w13:errorcluster)
  n152 = call "Close Module.vi"("error in"=w13, "Module Admin in"=w8) -> ("error out"=w15:errorcluster, "External Launch"=w2:bool, "Module Admin out"=w3:refnum<class "Delacor_lib_QMH_Module Admin.lvclass">)  [unwired: 7 in]
  n153 = Unregister For Events(event registration refnum=w7, error in=w15) -> (error out=w12:errorcluster)
  "error out" <- w12
  n154 = case "External Launch?" shown="True" w2 {
    tunnel: w12 -> [_ w291]
    frame False {
    }
    frame True {
      n155 = case shown="No Error" w291 {
        frame No Error {
          n156 = invoke on="Invoke Node" class="VI" method="FP.Close"() -> ()  [unwired: 3 in, 3 out]
        }
        frame Error {
          n157 = disable-structure shown="Default" {
            frame condition #0 (active) {
              n158 = invoke class="VI" method="FP.Open"("Activate"=TRUE ("Activate?")) -> ()  [unwired: 4 in, 5 out]
            }
            frame condition #1 {
              # "Don't show panel on error if running inside a built EXE."
            }
          }
        }
      }
    }
  }
  n159 = local write "Module Admin"(w3) -> ()
